vi "Arm.vi"(4 "Request type":T1=enum."User command", 6 "Init work":bool, 7 "Update period":dbl, 8 "error in (no error)":errorcluster, 9 "Last request":bool, 10 "Requester":string, 11 "RP I-V in":refnum<class "RP I-V.lvclass">) -> (0 "error out":errorcluster, 3 "RP I-V out":refnum<class "RP I-V.lvclass">)   [LabVIEW 2021, in "RP I-V.lvclass"]
uses:
  RP I-V.lvclass
  C:/GitHub/LabActor/Pulse Recorders/Pulse Recorder Actor/Pulse Recorder Actor.lvclass
  NHMFL_Core/Libraries/Red Pitaya/RP Core/Rep Pitaya I-V driver/RP I-V Driver.lvclass
  C:/GitHub/NHMFL_Core/Libraries/Instruments/Pulse Driver/Pulse Driver.lvclass
  NHMFL_Core/Libraries/Red Pitaya/RP Core/Rep Pitaya I-V driver/RP I-V Driver.lvclass/RP I-V Driver.ctl
  RP I-V.lvclass/RP I-V.ctl
  NHMFL_Core/Libraries/Red Pitaya/RP Core/Rep Pitaya I-V driver/Read Output waveform.vi
  Pulse Recorders/Pulse Recorder Actor/Read Pulse driver.vi
  Pulse Recorders/Pulse Recorder Actor/Write Pulse driver.vi
  Pulse Recorders/Pulse Recorder Actor/Pulse Recorder Actor.lvclass
  NHMFL_Core/Libraries/Instruments/Pulse Driver/Pulse Driver.lvclass
  C:/GitHub/NHMFL_Core/Libraries/Red Pitaya/Red Pitaya Digitizer/Red Pitaya Digitizer.lvclass
  C:/GitHub/NHMFL_Core/Libraries/Instruments/Pulse Driver/Lockin Digitizer Driver/Lockin Digitizer Driver.lvclass
  C:/GitHub/NHMFL_Core/Libraries/Instruments/Instrument Driver/Instrument Driver.lvclass
  C:/GitHub/NHMFL_Core/Libraries/Red Pitaya/RP Core/Rep Pitaya I-V driver/RP I-V Driver.lvclass
  Controllers/Process Controller/Request type.ctl
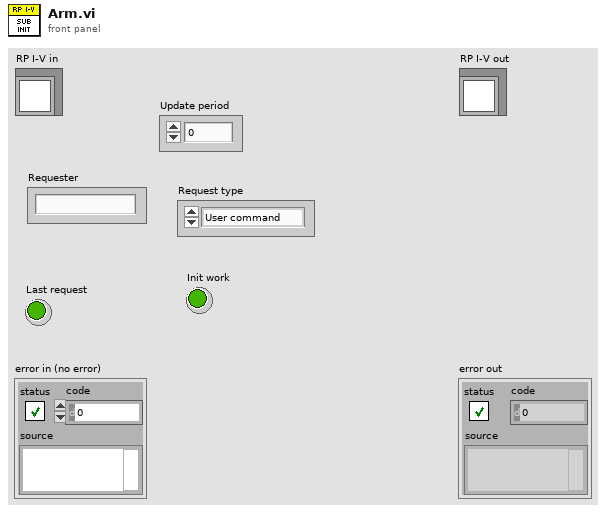
[diagram p1: front panel]
types:
  T1 = typedef "Request type.ctl" = enum16{"Process complete", "User command", "Auto-restart", "Error"}
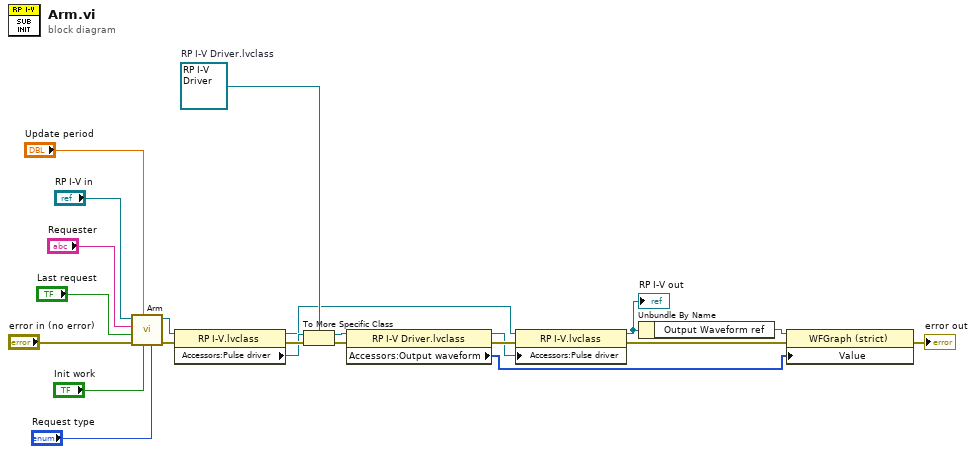
[diagram p0: block diagram]
diagram:
  w18 = refnum<class "RP I-V Driver.lvclass"> refnum  # RP I-V Driver.lvclass
  n1 = call-parent "Arm.vi"("Request type"="Request type", "Init work"="Init work", "Update period"="Update period", "error in (no error)"="error in (no error)", "Last request"="Last request", "Requester"="Requester", "Pulse Recorder Actor in"="RP I-V in") -> ("error out"=w15:errorcluster, "Pulse Recorder Actor out"=w11:refnum<class "RP I-V.lvclass">)  [unwired: 3 in]
  n2 = property class="RP I-V.lvclass"(reference=w11, error in=w15) -> (reference out=w12:refnum<class "RP I-V.lvclass">, error out=w20:errorcluster, "Accessors:Pulse driver"=w19:refnum<class "Pulse Driver.lvclass">)
  n3 = To More Specific Class(target class=w18, reference=w19, error in=w20) -> (specific class reference=w17:refnum<class "RP I-V Driver.lvclass">, error out=w16:errorcluster)
  n4 = property class="RP I-V Driver.lvclass"(reference=w17, error in=w16) -> (reference out=w13:refnum<class "RP I-V Driver.lvclass">, error out=w14:errorcluster, "Accessors:Output waveform"=w8:i16[])
  n5 = property class="RP I-V.lvclass"(reference=w12, error in=w14, "Accessors:Pulse driver"=w13) -> (reference out=w10:refnum<class "RP I-V.lvclass">, error out=w7:errorcluster)
  "RP I-V out" <- w10
  n6 = Unbundle By Name(w10) -> ("Output Waveform ref"=w9:refnum<vi>)
  n7 = property class="WFGraph (strict)"(reference=w9, error in=w7, "Value"=w8) -> (error out=→"error out":errorcluster)  [unwired: 1 out]
